vi "Robot Global Data.vi"() -> ()   [LabVIEW 2014]
doc: "This global VI can contain as many global variables as you need. Place a control on the panel, give it a good name. To read or write to it from a VI, drag the icon to the diagram of that VI. You can also drag from the project. Click on the node to change which global you access. You shouldn't have multiple locations writing to a global or it will cause a race-condition."
uses:
  <vilib>/Rock Robotics/WPI/Camera/WPI_CameraImageSize.ctl
  <vilib>/Rock Robotics/WPI/DriverStation/WPI_DriverStationRobotMode2.ctl
panel:
  in  "TapeMeasureTarget":dbl
  in  "TapeMeasureEncoder":dbl
  out "RollerSolenoidValue":bool
  in  "RollerMotorValue":dbl
  in  "TapeMeasure":dbl
  in  "CompressorAmperage":dbl
  out "CompressorState":bool
  in  "EncoderRight":dbl
  in  "EncoderLeft":dbl
  in  "BatteryVoltage":dbl
  in  "AutoStackState":T1(ring)
  in  "PIDCurrentState":T2(ring)
  out "PIDInPositionDwell":bool
  out "DriverGrabberControl":bool
  in  "StrafeSolenoid":bool
  in  "LoopTime":dbl
  in  "DriverReqPIDTarget":dbl
  out "DriverElevatorReset":bool
  out "GoatDetectorPhotoeye":bool
  out "DriverManualOverride":bool
  in  "DriverGripperSolenoid":bool
  out "AutoStackEnabled":bool
  out "AutoStackSolenoid":bool
  out "StackAllButton":bool
  out "AutoStackButton":bool
  in  "Joystick 1/SetRumble":dbl
  in  "Joystick 0/SetRumble":dbl
  in  "GripperSolenoid":bool
  in  "AmpLimit":dbl
  out "BottomOvertravel":bool
  out "TopOvertravel":bool
  in  "PIDInPosition":bool
  in  "GyroAngle":dbl
  in  "ElevatorAmperage":dbl
  in  "ZeroError":bool
  in  "ManualOutput":dbl
  in  "PIDOutput":dbl
  out "PIDEncoderReset":bool
  out "ElevatorReset":bool
  out "ElevatorManualOverride":bool
  out "Joystick 1/Buttons":bool[](array[boolean])
  out "Joystick 0/Buttons":bool[](array[boolean])
  out "Joystick 1/Axes":dbl[](array[numeric])
  out "Joystick 0/Axes":dbl[](array[numeric])
  out "PIDPhotoeye":bool
  in  "PIDTarget":dbl
  in  "PIDCurrent":dbl
  in  "ElevatorMotorValue":dbl
  in  "StrafeMotorValue":dbl
  in  "RightMotorValue":dbl
  in  "LeftMotorValue":dbl
  in  "Robot Mode":T3
  in  "image size":T4=enum."320x240"
  in  "Enable Vision":bool
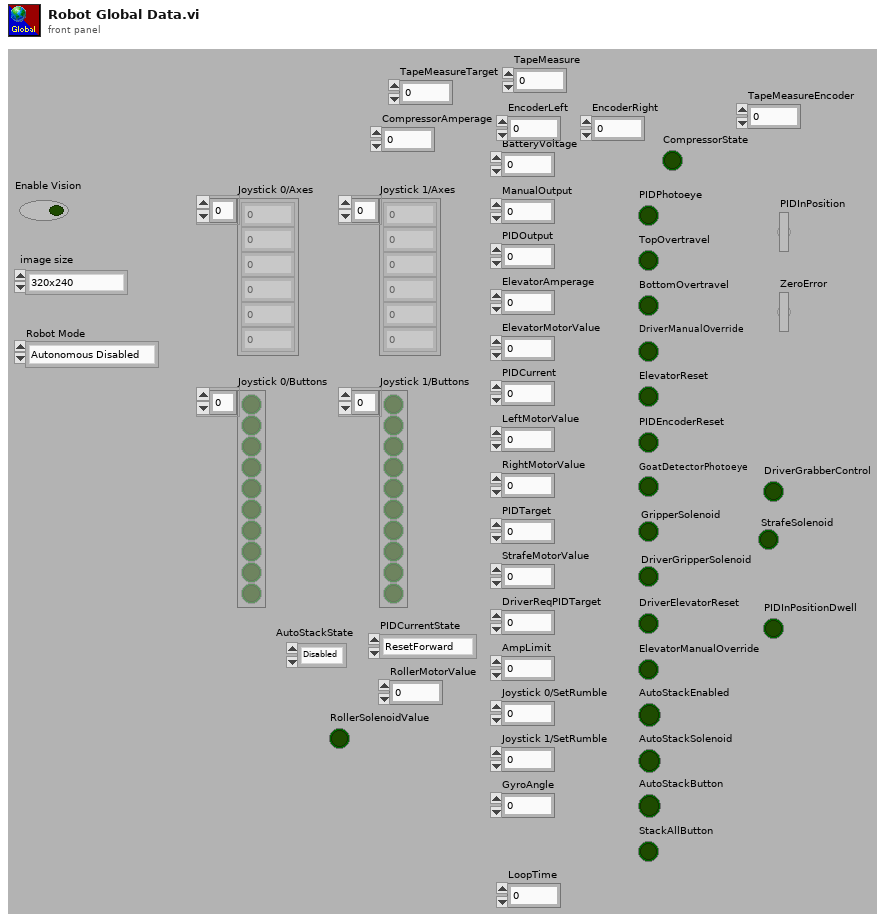
[diagram p1: front panel]
types:
  T1 = enum16{"Disabled", "Initialize", "CalcNewTarget", "Moving", "OpenArm", "CloseArm", "Reset"}
  T2 = enum16{"ResetForward", "ResetBack", "PIDControl", "ManualControl", "ZeroEncoderAndTarget", "AutoStack"}
  T3 = typedef "WPI_DriverStationRobotMode2.ctl" = enum16{"Autonomous Disabled", "Autonomous Enabled", "Teleop Disabled", "Teleop Enabled", "Disconnected", "Finish", "Test Disabled", "Test Enabled", "Emergency Stopped"}
  T4 = typedef "WPI_CameraImageSize.ctl" = enum16{"640x480", "320x240", "160x120", "Custom"}
diagram:
